vi "TxBegin_Core.vi"(8 "error in (no error)":errorcluster, 11 "DbConnection in":refnum<class "ORM_DBC_dotNet.lvclass">) -> (0 "error out":errorcluster, 3 "DbConnection out":refnum<class "ORM_DBC_dotNet.lvclass">)   [LabVIEW 2020, in "ORM_DBC_dotNet.lvlib" / "ORM_DBC_dotNet.lvclass"]
uses:
  ORM_DBC_dotNet.lvclass
  ORM_DBC_dotNet.lvclass/ORM_DBC_dotNet.ctl
  Read connection.vi
  Read transactions.vi
  Write connection.vi
  Write transactions.vi
  System.Data
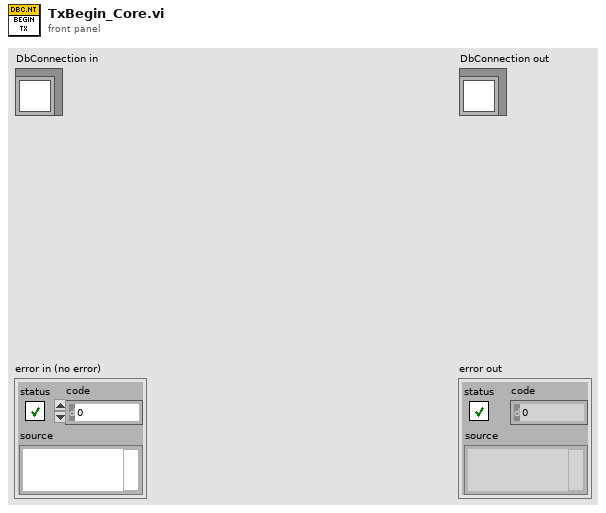
[diagram p1: front panel]
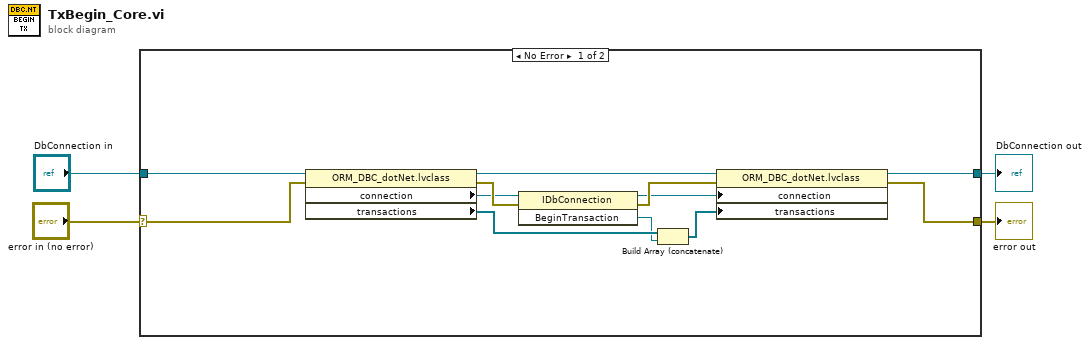
[diagram p0: block diagram]
diagram:
  n1 = case shown="No Error" "error in (no error)" {
    selector: "error in (no error)" -> [w15 w18]
    tunnel: [w14 w18] -> w3
    tunnel: [w16 w17] -> w1
    tunnel: "DbConnection in" -> [w13 w17]
    frame No Error {
      n2 = property class="ORM_DBC_dotNet.lvclass"(reference=w13, error in=w15) -> (reference out=w7:refnum<class "ORM_DBC_dotNet.lvclass">, error out=w11:errorcluster, "connection"=w10:refnum<k24>, "transactions"=w9:refnum<k24>[])
      n3 = invoke class="IDbConnection" method="BeginTransaction"(reference=w10, error in=w11) -> (reference out=w6:refnum<k24>, error out=w12:errorcluster, "BeginTransaction"=w8:refnum<k24>)  [unwired: 1 in]
      n4 = Build Array (concatenate)(w9, w8) -> (w5:refnum<k24>[])
      n5 = property class="ORM_DBC_dotNet.lvclass"(reference=w7, error in=w12, "connection"=w6, "transactions"=w5) -> (reference out=w16:refnum<class "ORM_DBC_dotNet.lvclass">, error out=w14:errorcluster)
    }
    frame Error {
    }
  }
  "error out" <- w3
  "DbConnection out" <- w1
